vi "Target Standard Logger.vi"(8 "Stop Command":bool, 10 "Incoming Data Array":dbl[](array[numeric]), 11 "Valid for Logging?":bool) -> (0 "Ok to Stop Logging Loop":bool)   [LabVIEW 2018, in "COBRA Logging Library.lvlib"]
uses:
  COBRA Logging Library.lvlib
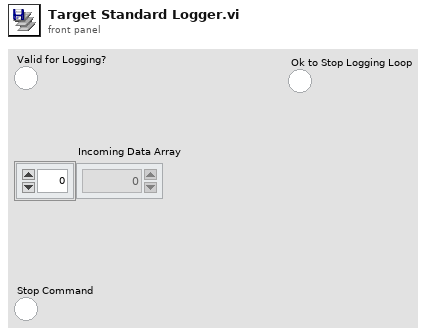
[diagram p1: front panel]
types:
  T1 = enum16{"Idle", "Accumulate", "Write Main", "Write Metadata"}
  T2 = typedef "COBRA Logging Library.lvlib/Target Logger States.ctl" = enum16{"Idle", "Accumulate", "Write Main", "Write Metadata"}
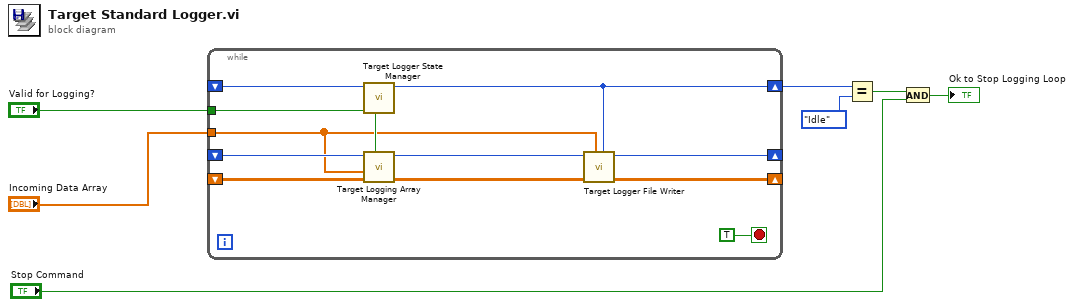
[diagram p0: block diagram]
diagram:
  n1 = while {
    tunnel: "Valid for Logging?" -> [w17]
    shift-right: [w11] -> w3
    shift-left: _ -> [w18]
    shift-right: [w15] -> _
    shift-left: _ -> [w13]
    shift-right: [w12] -> _
    shift-left: _ -> [w16]
    tunnel: "Incoming Data Array" -> [w8]
    stop <- TRUE stop-if-true
    n2 = call "Target Logger State Manager.vi"("Valid for Logging?"=w17, "Previous State"=w18) -> ("Current State"=w11:T2, "Preallocate Array?"=w9:bool)  [unwired: 8 in]
    n3 = call "Target Logging Array Manager.vi"("Allocate New Array"=w9, "Input Array"=w13, "Incoming Data Array"=w8, "Previous Index"=w16) -> ("Output Array"=w14:dbl[][], "Array Index to Write"=w10:i32)  [unwired: 6 in]
    n4 = call "Target Logger File Writer.vi"("State"=w11, "Incoming Data Array"=w8, "Input Array"=w14, "Array Index"=w10) -> ("Output Array"=w15:dbl[][], "Array Index Out"=w12:i32)  [unwired: 6 in]
  }
  n5 = Equal?(x=w3, y=T1."Idle") -> (x = y?=w2:bool)
  n6 = And(x=w2, y="Stop Command") -> (x .and. y?=→"Ok to Stop Logging Loop":bool)
